vi "MICS_ID Global.vi"() -> ()   [LabVIEW 2020]
panel:
  in  "MICS_ID":u32 format="%06x"
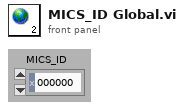
[diagram p1: front panel]
diagram:
